vi "Converter_search_input_unit_get_column.vi"(10 "unit to search for":i32, 11 "Unit conf cat. in":string[](array[string])) -> (3 "found in column number":i32)   [LabVIEW 2013]
doc: "Input is unboundled string array for selecting the unit category from application specific conversion settings cluster.\n\nOutput is column that the unit was found in, or -1 if not found.\n\nIf searched for unit#0 (not really valid), result not guaranteed."
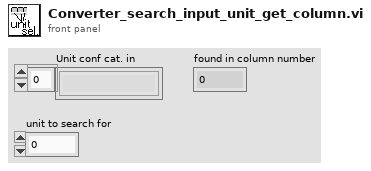
[diagram p1: front panel]
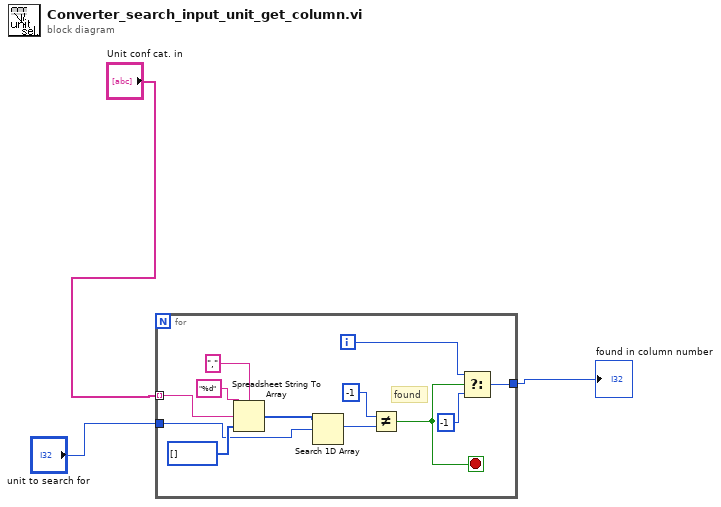
[diagram p0: block diagram]
diagram:
  n1 = for {
    tunnel: "Unit conf cat. in" -> [w13] mode=indexing
    tunnel: "unit to search for" -> [w10]
    tunnel: [w4] -> w3
    i -> [w6]
    stop <- w7 stop-if-true
    # "found"
    n2 = Spreadsheet String To Array(delimiter (Tab)=",", format string="%d", spreadsheet string=w13, array type (2D Dbl)=i32[] []) -> (array=w11:i32[])
    n3 = Search 1D Array(1D array=w11, element=w10) -> (index of element=w9:i32)  [unwired: 1 in]
    n4 = Not Equal?(x=-1, y=w9) -> (x != y?=w7:bool)
    n5 = Select(t=w6, s=w7, f=-1) -> (s? t:f=w4:i32)
  }
  "found in column number" <- w3
